vi "Lock LL Data (SubVI).vi"(11 "shoot":bool) -> (2 "Boolean":bool, 3 "Output cluster":T1)   [LabVIEW 2020]
panel:
  out "distance":dbl
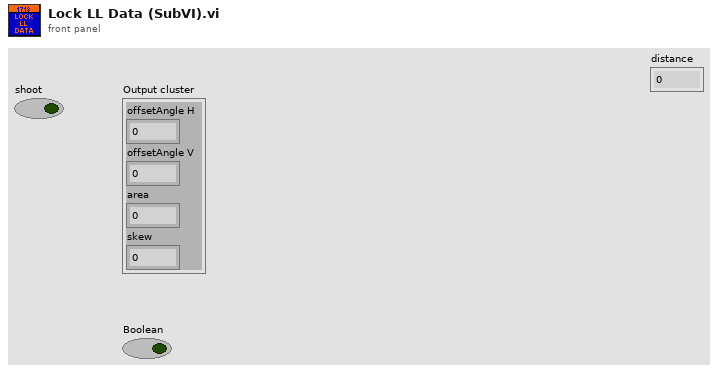
[diagram p1: front panel]
types:
  T1 = cluster{"offsetAngle H":dbl, "offsetAngle V":dbl, "area":dbl, "skew":dbl}
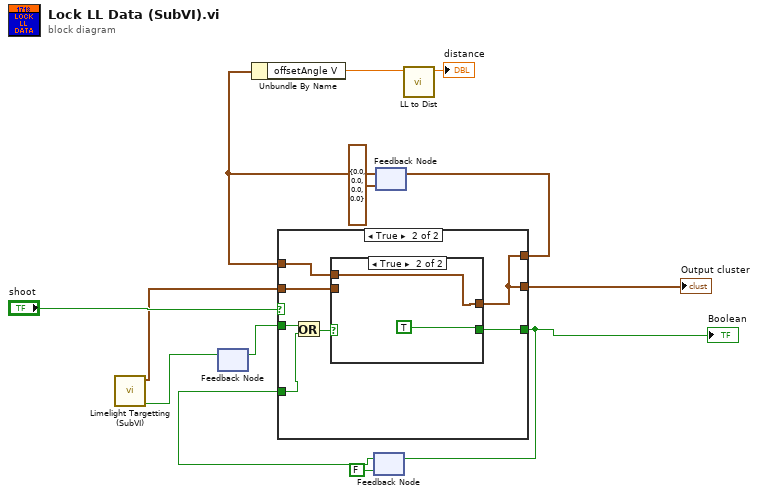
[diagram p0: block diagram]
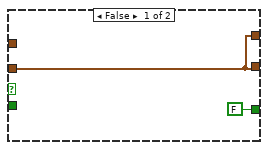
[diagram p2: hidden frame]
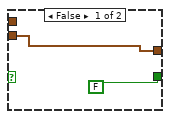
[diagram p3: hidden frame]
diagram:
  n1 = call "Limelight Targetting (SubVI).vi"() -> ("targetObtained"=w10:bool, "Output cluster"=w6:T1)  [unwired: 10 in]
  n2 = feedback #1() -> (w11:bool)  [unwired: 1 in]
  n3 = feedback-in #1(w10) -> ()
  n4 = feedback #2(FALSE) -> (w12:bool)
  n5 = feedback #3(T1 {"offsetAngle H"=0.0, "offsetAngle V"=0.0, "area"=0.0, "skew"=0.0} ("Output cluster")) -> (w3:T1)
  n6 = Unbundle By Name(w3) -> ("offsetAngle V"=w2:dbl)
  n7 = case shown="True" "shoot" {
    tunnel: w6 -> [w14 w22]
    tunnel: [w14 w21] -> w7
    tunnel: w11 -> [_ w19]
    tunnel: [w14 w21] -> w9
    tunnel: w3 -> [_ w20]
    tunnel: [FALSE w17] -> w13
    tunnel: w12 -> [_ w16]
    frame False {
    }
    frame True {
      n8 = Or(x=w19, y=w16) -> (x .or. y?=w18:bool)
      n9 = case shown="True" w18 {
        tunnel: [w24 w26] -> w21
        tunnel: w22 -> [w24 _]
        tunnel: w20 -> [_ w26]
        tunnel: [FALSE TRUE] -> w17
        frame False {
        }
        frame True {
        }
      }
    }
  }
  "Boolean" <- w13
  "Output cluster" <- w7
  n10 = feedback-in #2(w13) -> ()
  n11 = feedback-in #3(w9) -> ()
  n12 = call "LL to Dist.vi"("limelightV"=w2) -> ("distance"=→"distance":dbl)  [unwired: 10 in]
